vi "Engine_BuildDevPart.vi"(5 "FileInventory":T1[](array[typedef]) {"TargetType" items=["Relative to default installation directory"=68, "Root directory on first partition"=70, "Relative to directory table key"=82, "Absolute path to file"=65]}, 7 "EventStruct":T6, 8 "ErrIn":errorcluster, 10 "Project":refnum<vi>, 11 "IB_MSI.lvclass":refnum<class "IB_MSI.lvclass">) -> (0 "ErrOut":errorcluster)   [LabVIEW 2020, in "IB_MSI.lvclass"]
uses:
  <vilib>/AppBuilder/IB_Classes/MSI/IB_MSI.lvclass
  <vilib>/AppBuilder/IB_Classes/MSI/IB_MSI.lvclass/IB_MSI.ctl
  AppLibs/distkit/MDF/NI_MDF.lvlib
  AppLibs/distkit/MDF/NIMdf.llb/MDFBDPSetBitnessModeType.ctl
  <vilib>/AppBuilder/IB_Classes/Installer/Installer.lvclass
  <vilib>/AppBuilder/IB_Classes/Destination/IB_Destination.lvclass
  e:/builds/penguin/labview/branches/2020/dev/dist/vi.lib/AppBuilder/IB_Classes/Installer/Installer.lvclass
  e:/builds/penguin/labview/branches/2020/dev/dist/vi.lib/AppBuilder/IB_Classes/MSI/IB_MSI.lvclass
  <resource>/Framework/Providers/API/mxLvBuildNewJob.ctl
  <resource>/Framework/Providers/API/mxLvBuildNewItem.ctl
  AppLibs/distkit/MDF/NIMdf.llb/MDFBDPAddFilePathType.ctl
  <resource>/Framework/Providers/Builds/Installer/CDK_sTypeDef_DevPartInventory.ctl
  <resource>/Framework/Providers/Builds/Installer/CDK_sTypeDef_DevPartShortcut.ctl
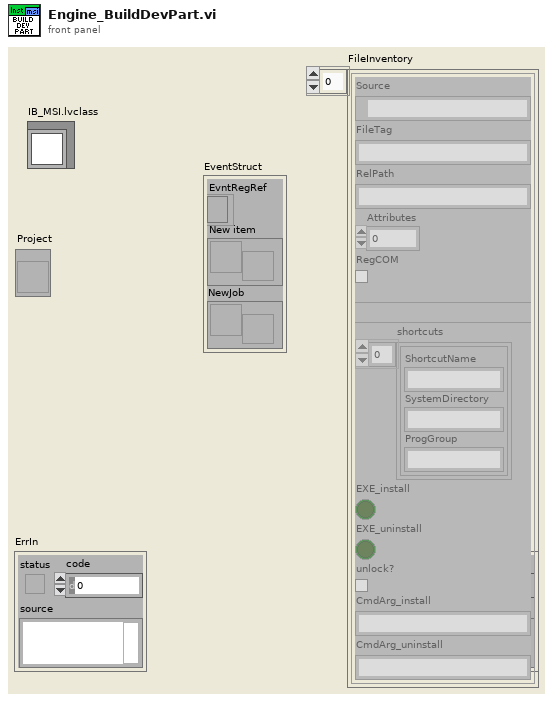
[diagram p1: front panel]
types:
  T1 = typedef "CDK_sTypeDef_DevPartInventory.ctl" = cluster{"Source":path, "FileTag":string, "RelPath":string, "Attributes":i32, "RegCOM":bool, "TargetType":T2, "shortcuts":T3[], "EXE_install":bool, "EXE_uninstall":bool, "unlock?":bool, "CmdArg_install":string, "CmdArg_uninstall":string}
  T2 = typedef "NI_MDF.lvlib/MDFBDPAddFilePathType.ctl" = i32
  T3 = typedef "CDK_sTypeDef_DevPartShortcut.ctl" = cluster{"ShortcutName":string, "SystemDirectory":string, "ProgGroup":string}
  T4 = typedef "mxLvBuildNewItem.ctl" = refnum<user-event>
  T5 = typedef "mxLvBuildNewJob.ctl" = refnum<user-event>
  T6 = cluster{"EvntRegRef":refnum<event-registration>, "New item":T4, "NewJob":T5}
  T7 = typedef "NI_MDF.lvlib/MDFBDPSetBitnessModeType.ctl" = i32
  T8 = typedef "IB_Installer.ctl" = cluster{"Destination":refnum<class "IB_Destination.lvclass">[], "Source":refnum<class "IB_Source.lvclass">[], "buildObject":T9, "defaultDir":string, "platform":string, "author":string, "productName":string, "buildSpecName":string, "hide":bool, "requireLVDevSys":bool, "autoIncrement":bool, "includeError":bool, "readmeID":string, "buildLocation":path, "readmePath":path, "mediaSize":u16, "language":T10, "productVersion":T11, "preview":bool, "programmatic":bool, "progressBarEvents":T12, "userLog_Path":path, "shortcutAddresses":T14[], "EXE_Install Address":string, "EXE_Uninstall Address":string, "additional NIPaths":refnum<class "Dest_NI_NIPath.lvclass">[], "web service itemIDs":string[], "installerName":string}
  T9 = typedef "ItemRef.ctl" = u64
  T10 = typedef "CDK_sTypeDef_Languages.ctl" = u16
  T11 = typedef "CDK_sTypeDef_ProductVersion.ctl" = cluster{"Major":u8, "Minor":u8, "Update":u16}
  T12 = typedef "provcom_ProgressBar_Events.ctl" = cluster{"newJob":refnum<user-event>, "newItem":refnum<user-event>, "errorMsg":T13, "cancel":refnum<user-event>}
  T13 = typedef "mxLvBuildError.ctl" = refnum<user-event>
  T14 = typedef "CDK_sTypeDef_ShortcutAddress.ctl" = cluster{"file":string, "shortcut":string}
  T15 = typedef "IB_MSI.ctl" = cluster{"upgradeCode":string, "distID":string, "windowMessage":string, "windowTitle":string, "arpPhone":string, "arpContact":string, "arpURL":string, "arpCompany":string, "licenseID":string, "licensePath":path, "welcomeImageID":string, "welcomeImagePath":path, "bannerImageID":string, "bannerImagePath":path, "osCheck":i32, "msiFileName":string, "cabFileName":string, "hwOption":T16, "hwPath":path, "regGroup":refnum<class "IB_RegGroup.lvclass">[], "regDest":refnum<class "IB_RegDest.lvclass">[], "selectedDists":refnum<class "IB_DistPart.lvclass">[], "installedDists":refnum<class "IB_DistPart.lvclass">[], "postInstallSteps":refnum<class "IB_Post_Install_Step.lvclass">[], "preUninstallSteps":refnum<class "IB_Post_Install_Step.lvclass">[], "winsec.certificate":string, "winsec.timestamp":string, "winsec.description":string, "autoselect drivers":bool, "hide non-runtimes":bool}
  T16 = typedef "CDK_sTypeDef_HWImportOption.ctl" = enum16{"<none>", "Merge", "Replace", "Dialog"}
  T17 = typedef "CDK_sTypeDef_AppBitness.ctl" = enum16{"invalid", "32-bit", "64-bit"}
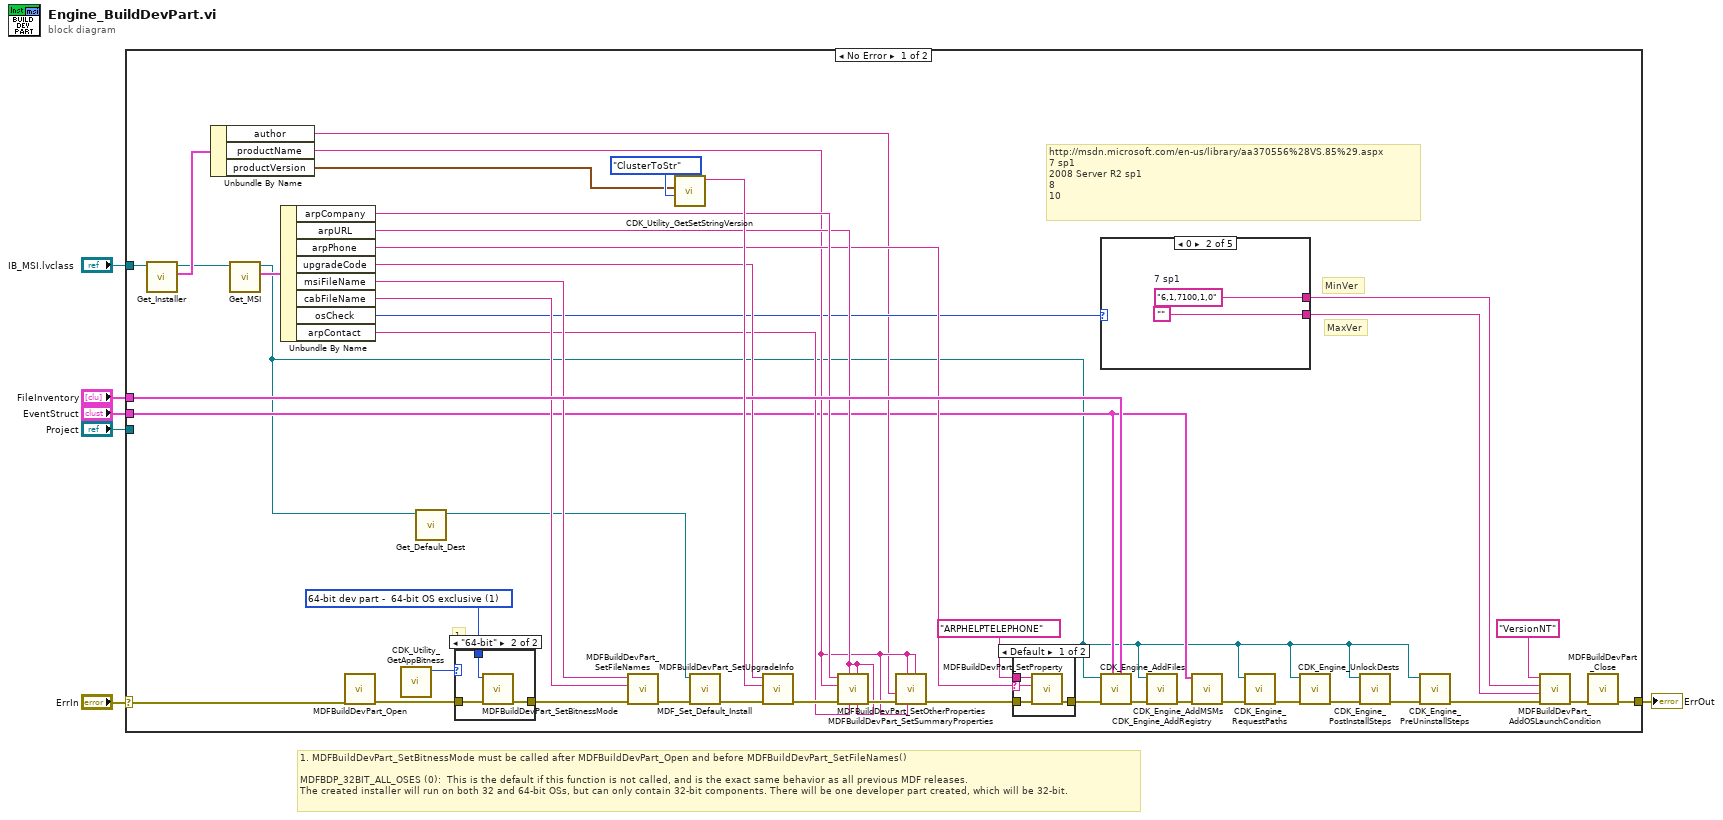
[diagram p0: block diagram]
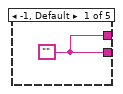
[diagram p4: hidden frame]
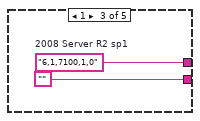
[diagram p5: hidden frame]
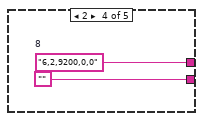
[diagram p6: hidden frame]
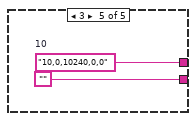
[diagram p7: hidden frame]
diagram:
  # "1. MDFBuildDevPart_SetBitnessMode must be called after MDFBuildDevPart_Open and before MDFBuildDevPart_SetFileNames()\n\nMDFBDP_32BIT_ALL_OSES (0):  This is the default if this function is not called, and is the exact same behavior as all previous MDF releases.\nThe created installer will run on both 32 and 64-bit OSs, but can only contain 32-bit components. There will be one developer part created, which will be 32-bit."
  n1 = case shown="No Error" "ErrIn" {
    selector: "ErrIn" -> [w44 w70]
    tunnel: [w43 w70] -> w5
    tunnel: "Project" -> [_ _]
    tunnel: "EventStruct" -> [w16 _]
    tunnel: "FileInventory" -> [w47 _]
    tunnel: "IB_MSI.lvclass" -> [w30 _]
    frame No Error {
      w32 = T7 1 items=["32-bit dev part - run on all OSes", "64-bit dev part -  64-bit OS exclusive", "32/64-bit hybrid - run on all OSes"] ("bitness mode type (for dev part)")
      # "http://msdn.microsoft.com/en-us/library/aa370556%28VS.85%29.aspx\n7 sp1\n2008 Server R2 sp1\n8\n10"
      # "1."
      # "MaxVer"
      # "MinVer"
      n2 = call <vilib>:"Get_Installer.vi"("Installer in"=w30) -> ("data"=w29:T8, "Installer out"=w17:refnum<class "IB_MSI.lvclass">)  [unwired: 1 in, 8 out]
      n3 = Unbundle By Name(w29) -> ("author"=w18:string, "productName"=w23:string, "productVersion"=w24:T11)
      n4 = call <vilib>:"Get_MSI.vi"("IB_MSI in"=w17) -> ("data"=w31:T15, "IB_MSI out"=w9:refnum<class "IB_MSI.lvclass">)  [unwired: 1 in, 8 out]
      n5 = Unbundle By Name(w31) -> ("arpCompany"=w28:string, "arpURL"=w27:string, "arpPhone"=w26:string, "upgradeCode"=w25:string, "msiFileName"=w22:string, "cabFileName"=w21:string, "osCheck"=w20:i32, "arpContact"=w19:string)
      n6 = call "MDFBuildDevPart_Open.vi"("error in (no error)"=w44) -> ("error out"=w34:errorcluster)  [unwired: 10 out]
      n7 = call <resource>:"CDK_Utility_GetAppBitness.vi"() -> ("app bitness"=w35:T17)  [unwired: 11 out]
      n8 = call <vilib>:"Get_Default_Dest.vi"("Installer in"=w9) -> ("IB_Destination.lvclass"=w10:refnum<class "IB_Destination.lvclass">)  [unwired: 1 in, 9 out]
      n9 = case shown="\"64-bit\"" w35 {
        tunnel: w34 -> [w52 w54]
        tunnel: [w52 w55] -> w33
        tunnel: w32 -> [_ w53]
        frame "32-bit", Default {
        }
        frame "64-bit" {
          n10 = call "MDFBuildDevPart_SetBitnessMode.vi"("error in (no error)"=w54, "bitness mode type (for dev part)"=w53) -> ("error out"=w55:errorcluster)  [unwired: 9 out]
        }
      }
      n11 = call "MDFBuildDevPart_SetFileNames.vi"("error in (no error)"=w33, ".cab file name"=w21, ".msi file name"=w22) -> ("error out"=w12:errorcluster)  [unwired: 8 out]
      n12 = call <resource>:"CDK_Utility_GetSetStringVersion.vi"("Action"=enum16{"ClusterToStr", "StrToCluster"}."ClusterToStr", "ProductVersionIn"=w24) -> ("VersionStringOut"=w48:string)  [unwired: 2 in, 7 out]
      n13 = call-dynamic "MDF_Set_Default_Install.vi"("error in (no error)"=w12, "IB_Destination in"=w10) -> ("error out"=w11:errorcluster)  [unwired: 9 out]
      n14 = call "MDFBuildDevPart_SetUpgradeInfo.vi"("error in (no error)"=w11, "product version"=w48, "upgrade code"=w25) -> ("error out"=w49:errorcluster)  [unwired: 8 out]
      n15 = call "MDFBuildDevPart_SetOtherProperties.vi"("ARP help link"=w27, "ARP URL product update info"=w27, "ARP contact"=w19, "ARP URL info about"=w27, "error in (no error)"=w49, "project name"=w23, "manufacturer"=w28) -> ("error out"=w50:errorcluster)  [unwired: 1 in, 3 out]
      n16 = call "MDFBuildDevPart_SetSummaryProperties.vi"("summary title"=w23, "summary application name"=w23, "summary subject"=w23, "error in (no error)"=w50, "summary author"=w18) -> ("error out"=w38:errorcluster)  [unwired: 3 in, 3 out]
      n17 = case shown="Default" w26 {
        selector: w26 -> [w57 _]
        tunnel: w38 -> [w59 w60]
        tunnel: [w58 w60] -> w37
        tunnel: "ARPHELPTELEPHONE" ("OS family") -> [w56 _]
        frame Default {
          n18 = call "MDFBuildDevPart_SetProperty.vi"("error in (no error)"=w59, "property value"=w57, "property name"=w56) -> ("error out"=w58:errorcluster)  [unwired: 8 out]
        }
        frame "" {
        }
      }
      n19 = case shown="0" w20 {
        tunnel: [w61 w63 w65 w67 w69] -> w40
        tunnel: [w61 "" "" "" ""] -> w39
        frame -1, Default {
          w61 = ""
        }
        frame 0 {
          w63 = "6,1,7100,1,0"  # 7 sp1
        }
        frame 1 {
          w65 = "6,1,7100,1,0"  # 2008 Server R2 sp1
        }
        frame 2 {
          w67 = "6,2,9200,0,0"  # 8
        }
        frame 3 {
          w69 = "10,0,10240,0,0"  # 10
        }
      }
      n20 = call <resource>:"CDK_Engine_AddFiles.vi"("FileInventory"=w47, "EventStruct"=w16, "ErrIn"=w37, "IB_MSI.lvclass"=w9) -> ("ErrOut"=w46:errorcluster)  [unwired: 7 out]
      n21 = call <resource>:"CDK_Engine_AddRegistry.vi"("ErrIn"=w46, "IB_MSI.lvclass"=w9) -> ("ErrOut"=w45:errorcluster)  [unwired: 9 out]
      n22 = call <resource>:"CDK_Engine_AddMSMs.vi"("ErrIn"=w45, "EventStruct"=w16) -> ("ErrOut"=w15:errorcluster)  [unwired: 1 in, 8 out]
      n23 = call <resource>:"CDK_Engine_RequestPaths.vi"("ErrIn"=w15, "IB_MSI.lvclass"=w9) -> ("ErrOut"=w14:errorcluster)  [unwired: 9 out]
      n24 = call <resource>:"CDK_Engine_UnlockDests.vi"("ErrIn"=w14, "IB_MSI.lvclass"=w9) -> ("ErrOut"=w13:errorcluster)  [unwired: 9 out]
      n25 = call <resource>:"CDK_Engine_PostInstallSteps.vi"("ErrIn"=w13, "IB_MSI.lvclass"=w9) -> ("ErrOut"=w8:errorcluster)  [unwired: 9 out]
      n26 = call <resource>:"CDK_Engine_PreUninstallSteps.vi"("ErrIn"=w8, "IB_MSI.lvclass"=w9) -> ("ErrOut"=w7:errorcluster)  [unwired: 9 in]
      n27 = call "MDFBuildDevPart_AddOSLaunchCondition.vi"("error in (no error)"=w7, "version max"=w39, "version min"=w40, "OS family"="VersionNT") -> ("error out"=w42:errorcluster)  [unwired: 1 in, 6 out]
      n28 = call "MDFBuildDevPart_Close.vi"("error in (no error)"=w42) -> ("error out"=w43:errorcluster)  [unwired: 10 out]
    }
    frame Error {
    }
  }
  "ErrOut" <- w5
